vi "XY Graph Set Style of Selected Plots.vi"(8 "Error In":errorcluster, 9 "Plot Style":T2={"Plot Style"=enum."unchanged", "Histogram Type"=enum."Left Bound", "Line Tickness"=enum."unchanged", "Line Style"=enum."unchanged", "Point Style"=enum."Small Filled Square", "Line Color"=0, "Point Color"=0, "Anti-aliased"=FALSE, "Line Color Chooser"=enum."unchanged", "Point Color Chooser"=enum."unchanged", "Line Color List"="", "Point Color List"=""}, 11 "XYGraph Ref":T1) -> (0 "Error Out":errorcluster, 1 "Message":string, 3 "XYGraph Ref":T1, 5 "Graph Caption":string)   [LabVIEW 2019, in "XY Graph Add-Ons.lvlib"]
uses:
  XY Graph Add-Ons.lvlib
  XY Graph Refnum.ctl
  Plot Style 3.ctl
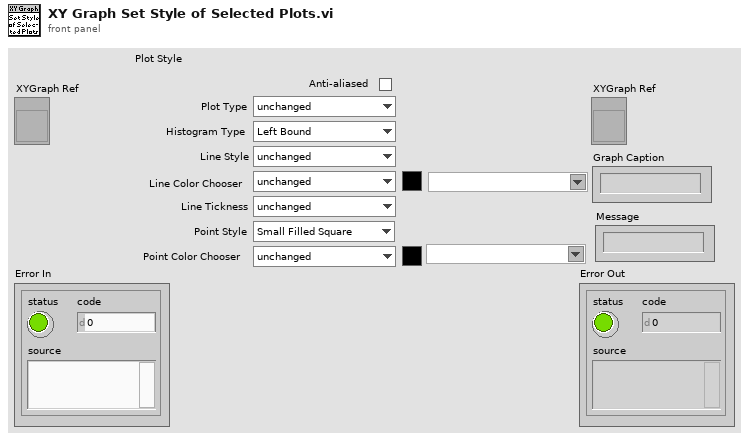
[diagram p1: front panel]
types:
  T1 = typedef "XY Graph Add-Ons.lvlib/XY Graph Refnum.ctl" = refnum<vi>
  T2 = typedef "Plot Style 3.ctl" = cluster{"Plot Style":enum16{"unchanged", "Line", "Symbol", "Line + Symbol", "Histogram", "Histogram + Symbol"}, "Histogram Type":enum16{"unchanged", "Left Bound", "Center", "Right Bound"}, "Line Tickness":enum16{"unchanged", "Thin", "1 pixel", "2 pixel", "3 pixel", "4 pixel", "5 pixel"}, "Line Style":enum16{"unchanged", "Plain", "Long Dash", "Short Dash", "Long-Short Dash", "Long-Short-Short Dash"}, "Point Style":enum16{"unchanged", "None", "Empty Circle", "Filled Circle", "Thick Circle", "Dotted Circle", "Empty Square", "Filled Square", "Thick Square", "Dotted Square", "Small Filled Square", "Dot", "Cross", "Tiny Cross", "Large X", "Small x", "Diamond", "Small Empty Square"}, "Line Color":u32, "Point Color":u32, "Anti-aliased":bool, "Line Color Chooser":enum16{"unchanged", "Color Box", "Color List"}, "Point Color Chooser":enum16{"unchanged", "Color Box", "Color List"}, "Line Color List":string, "Point Color List":string}
  T3 = typedef "Single Plot Style 2.ctl" = cluster{"Plot Style":enum16{"unchanged", "Line", "Symbol", "Line + Symbol", "Histogram", "Histogram + Symbol"}, "Histogram Type":enum16{"unchanged", "Left Bound", "Center", "Right Bound"}, "Line Tickness":enum16{"unchanged", "Thin", "1 pixel", "2 pixel", "3 pixel", "4 pixel", "5 pixel"}, "Line Style":enum16{"unchanged", "Plain", "Long Dash", "Short Dash", "Long-Short Dash", "Long-Short-Short Dash"}, "Point Style":enum16{"unchanged", "None", "Empty Circle", "Filled Circle", "Thick Circle", "Dotted Circle", "Empty Square", "Filled Square", "Thick Square", "Dotted Square", "Small Filled Square", "Dot", "Cross", "Tiny Cross", "Large X", "Small x", "Diamond", "Small Empty Square"}, "Line Color":u32, "Line Color defined?":bool, "Point Color":u32, "Point Color defined?":bool, "Anti-aliased":bool}
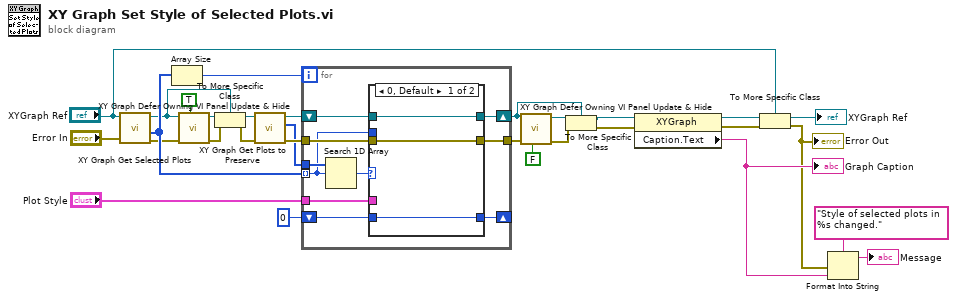
[diagram p0: block diagram]
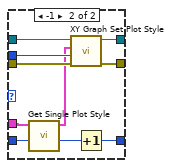
[diagram p2: hidden frame]
diagram:
  n1 = call "XY Graph Get Selected Plots.vi"("error in (no error)"="Error In", "XYGraph in"="XYGraph Ref") -> ("error out"=w25:errorcluster, "Selected Plots"=w29:i32[], "XYGraph out"=w13:T1)  [unwired: 5 in, 2 out]
  n2 = Array Size(array=w29) -> (size(s)=w28:i32)
  n3 = call "XY Graph Defer Owning VI Panel Update & Hide.vi"("Defer Owning Panel Update"=TRUE, "error in (no error)"=w25, "XY Graph Refnum in"=w13) -> ("error out"=w12:errorcluster)  [unwired: 7 in, 1 out]
  n4 = To More Specific Class(target class=w13, reference=w13, error in=w12) -> (specific class reference=w6:T1, error out=w5:errorcluster)
  n5 = call "XY Graph Get Plots to Preserve.vi"("Error In"=w5, "XYGraph in"=w6) -> ("Error Out"=w4:errorcluster, "Preserved Plots"=w2:i32[], "XYGraph out"=w3:T1)  [unwired: 6 in, 1 out]
  n6 = for {
    N: w28 -> [_]
    tunnel: w2 -> [w35]
    tunnel: w29 -> [w34] mode=indexing
    tunnel: "Plot Style" -> [w38]
    tunnel: w4 -> [w37]
    tunnel: [w36] -> w23
    shift-right: [w32] -> w9
    shift-left: w3 -> [w33]
    shift-right: [w30] -> _
    shift-left: 0 -> [w31]
    n7 = Search 1D Array(1D array=w35, element=w34) -> (index of element=w39:i32)  [unwired: 1 in]
    n8 = case shown="0, Default" w39 {
      tunnel: w34 -> [_ w47]
      tunnel: w33 -> [w41 w51]
      tunnel: w38 -> [_ w50]
      tunnel: w37 -> [w42 w49]
      tunnel: [w42 w48] -> w36
      tunnel: w31 -> [w40 w44]
      tunnel: [w41 w45] -> w32
      tunnel: [w40 w43] -> w30
      frame 0, Default {
      }
      frame -1 {
        n9 = call "Get Single Plot Style.vi"("index"=w44, "Plot Style in"=w50) -> ("Plot Style out"=w46:T3)  [unwired: 8 in, 1 out]
        n10 = call "XY Graph Set Plot Style.vi"("Error In"=w49, "Plot Index (0)"=w47, "Single Plot Style"=w46, "XY Graph Refnum in"=w51) -> ("Error Out"=w48:errorcluster, "XY Graph Refnum out"=w45:refnum<vi>)  [unwired: 6 in]
        n11 = Increment(x=w44) -> (x+1=w43:i32)
      }
    }
  }
  n12 = call "XY Graph Defer Owning VI Panel Update & Hide.vi"("Defer Owning Panel Update"=FALSE, "error in (no error)"=w23, "XY Graph Refnum in"=w9) -> ("error out"=w8:errorcluster, "XY Graph Refnum out"=w11:refnum<vi>)  [unwired: 7 in]
  n13 = To More Specific Class(target class=w9, reference=w11, error in=w8) -> (specific class reference=w10:refnum<vi>, error out=w7:errorcluster)
  n14 = property class="XYGraph"(reference=w10, error in=w7) -> (reference out=w18:refnum<vi>, error out=w20:errorcluster, "Caption.Text"=w16:string)
  "Graph Caption" <- w16
  n15 = To More Specific Class(target class="XYGraph Ref", reference=w18, error in=w20) -> (specific class reference=→"XYGraph Ref":T1, error out=w14:errorcluster)
  "Error Out" <- w14
  n16 = Format Into String(format string="Style of selected plots in %s changed.", error in=w14, w16) -> (resulting string=→"Message":string)  [unwired: 1 in, 1 out]
